vi "AssignAndCount60_2Ch_AreaOut.vi"(7 "Area bits in":bool[](array[boolean])=[FALSE, FALSE, FALSE, FALSE, FALSE, FALSE, FALSE, FALSE, FALSE, FALSE, FALSE, FALSE, FALSE, FALSE, FALSE, FALSE, FALSE, FALSE, FALSE, FALSE, FALSE, FALSE, FALSE, FALSE, FALSE, FALSE, FALSE, FALSE, FALSE, FALSE, FALSE, FALSE, FALSE, FALSE, FALSE, FALSE, FALSE, FALSE, FALSE, FALSE, FALSE, FALSE, FALSE, FALSE, FALSE, FALSE, FALSE, FALSE, FALSE, FALSE, FALSE, FALSE, FALSE, FALSE, FALSE, FALSE, FALSE, FALSE, FALSE, FALSE], 8 "PMT bits Ch2 in":bool[](array[boolean])=[FALSE, FALSE, FALSE, FALSE, FALSE, FALSE, FALSE, FALSE, FALSE, FALSE, FALSE, FALSE, FALSE, FALSE, FALSE, FALSE, FALSE, FALSE, FALSE, FALSE, FALSE, FALSE, FALSE, FALSE, FALSE, FALSE, FALSE, FALSE, FALSE, FALSE, FALSE, FALSE, FALSE, FALSE, FALSE, FALSE, FALSE, FALSE, FALSE, FALSE, FALSE, FALSE, FALSE, FALSE, FALSE, FALSE, FALSE, FALSE, FALSE, FALSE, FALSE, FALSE, FALSE, FALSE, FALSE, FALSE, FALSE, FALSE, FALSE, FALSE], 9 "PMT bits Ch1 in":bool[](array[boolean])=[FALSE, FALSE, FALSE, FALSE, FALSE, FALSE, FALSE, FALSE, FALSE, FALSE, FALSE, FALSE, FALSE, FALSE, FALSE, FALSE, FALSE, FALSE, FALSE, FALSE, FALSE, FALSE, FALSE, FALSE, FALSE, FALSE, FALSE, FALSE, FALSE, FALSE, FALSE, FALSE, FALSE, FALSE, FALSE, FALSE, FALSE, FALSE, FALSE, FALSE, FALSE, FALSE, FALSE, FALSE, FALSE, FALSE, FALSE, FALSE, FALSE, FALSE, FALSE, FALSE, FALSE, FALSE, FALSE, FALSE, FALSE, FALSE, FALSE, FALSE], 10 "Photon counters area 2 in":cluster{u16, u16}, 11 "Photon counters area 1 in":cluster{u16, u16}) -> (2 "Photon counters area 2 out":cluster{u16, u16}, 3 "Photon counters area 1 out":cluster{u16, u16})   [LabVIEW 2012]
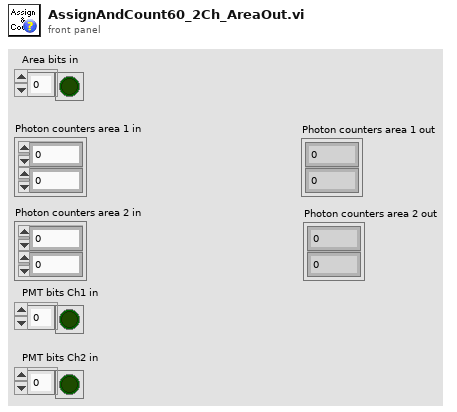
[diagram p1: front panel]
types:
  T1 = cluster{"New high count":u16, "New high count":u16}
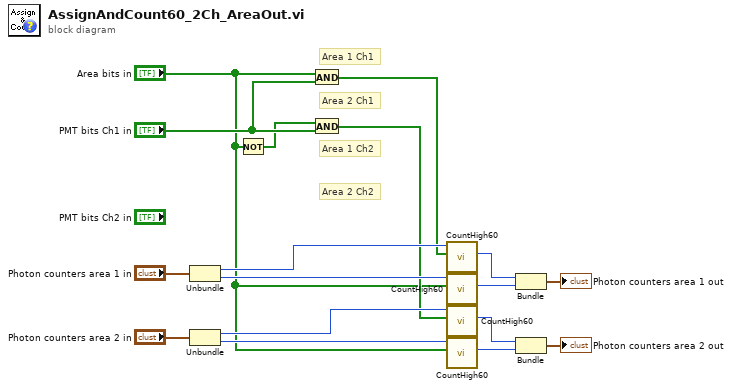
[diagram p0: block diagram]
diagram:
  # "Area 2 Ch2"
  # "Area 1 Ch2"
  # "Area 2 Ch1"
  # "Area 1 Ch1"
  n1 = Unbundle("Photon counters area 1 in") -> (w14:u16, w11:u16)
  n2 = Unbundle("Photon counters area 2 in") -> (w13:u16, w10:u16)
  n3 = Not(x="Area bits in") -> (.not. x?=w2:bool[])
  n4 = And(x="Area bits in", y="PMT bits Ch1 in") -> (x .and. y?=w12:bool[])
  n5 = And(x=w2, y="PMT bits Ch1 in") -> (x .and. y?=w3:bool[])
  n6 = call "CountHigh60.vi"("60bit input"=w12, "Previous high count"=w14) -> ("New high count"=w9:u16)  [unwired: 9 in]
  n7 = call "CountHigh60.vi"("60bit input"="Area bits in", "Previous high count"=w11) -> ("New high count"=w8:u16)  [unwired: 9 in]
  n8 = call "CountHigh60.vi"("60bit input"=w3, "Previous high count"=w13) -> ("New high count"=w7:u16)  [unwired: 9 in]
  n9 = call "CountHigh60.vi"("60bit input"="Area bits in", "Previous high count"=w10) -> ("New high count"=w6:u16)  [unwired: 9 in]
  n10 = Bundle("New high count"=w9, "New high count"=w8) -> (→"Photon counters area 1 out":T1)  [unwired: 1 in]
  n11 = Bundle("New high count"=w7, "New high count"=w6) -> (→"Photon counters area 2 out":T1)  [unwired: 1 in]
